vi "basic-reception.vi"(0 "Digital in":refnum<vi>, 1 "Cluster 5":T1, 2 "Lickometer":refnum<vi>, 3 "reference in":refnum<vi>, 5 "relative seconds":dbl, 7 "Cluster in":T2, 9 "Current Number Reception Licks":i32, 11 "Period":i64, 12 "Numeric 2":dbl, 13 "Numeric":dbl, 14 "Min Licks":i32) -> (4 "Cluster 4":T1, 6 "Cluster out":T2)   [LabVIEW 2015]
uses:
  <vilib>/Platform/TimedLoop/XDataNode/wakeup.ctl
  <vilib>/Platform/TimedLoop/XDataNode/XDNodeRunTimeDep.lvlib
  <vilib>/Platform/TimedLoop/XDataNode/nitl_modes.ctl
  <vilib>/Platform/TimedLoop/XDataNode/timing_clust.ctl
  <vilib>/platform/TimedLoop/XDataNode/XDataNode.xnode
  Device/Methods/Lickometer-Read.vi
  Rack/Methods/Rack-Refresh.vi
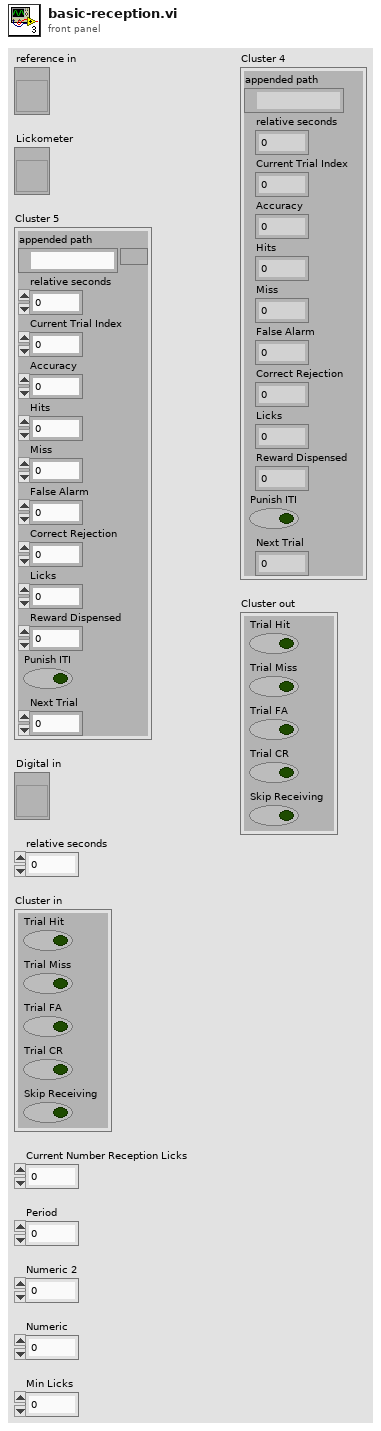
[diagram p1: front panel]
types:
  T1 = cluster{"appended path":path, "relative seconds":dbl, "Current Trial Index":i32, "Accuracy":dbl, "Hits":i32, "Miss":i32, "False Alarm":i32, "Correct Rejection":i32, "Licks":i32, "Reward Dispensed":dbl, "Punish ITI":bool, "Next Trial":i32}
  T2 = cluster{"Trial Hit":bool, "Trial Miss":bool, "Trial FA":bool, "Trial CR":bool, "Skip Receiving":bool}
  T3 = typedef "XDNodeRunTimeDep.lvlib/timing_clust.ctl" = cluster{"Expected End [f-1]":u64, "Actual End [f-1]":u64, "Finished Late? [f-1]":bool, "Expected End [i-1]":u64, "Actual End [i-1]":u64, "Finished Late? [i-1]":bool, "Expected Start [i]":u64, "Actual Start [i]":u64, "Expected Start [f]":u64, "Actual Start [f]":u64, "Source Name":string, "Structure Name":string, "Period":i64, "Deadline":i64, "Offset":i64, "Start":i64, "Priority":i32, "Timeout":i32, "Mode":T4, "Wakeup Reason":T5, "Error":errorcluster, "Source Type":string, "Secondary Source Type":string, "Global End Time":u64, "Global Start Time":u64, "Frame Duration":u64, "Iteration Duration":u64, "Assigned CPU":i32, "I/O Scan Engine Mode":u32}
  T4 = typedef "XDNodeRunTimeDep.lvlib/nitl_modes.ctl" = enum32{"No Change", "Process missed periods, maintain original phase", "Discard missed periods, maintain original phase", "Process missed periods, ignore original phase", "Discard missed periods, ignore original phase"}
  T5 = typedef "XDNodeRunTimeDep.lvlib/wakeup.ctl" = enum32{"Normal", "Aborted", "Asynchronous wakeup", "Timing source error", "Timed loop error", "Timeout"}
  T6 = typedef "InputData cluster.ctl" = cluster{"DigitalInput":T7}
  T7 = typedef "DigitalInput-DataCluster.ctl" = cluster{"Falling":bool[], "Rising":bool[], "State":bool[]}
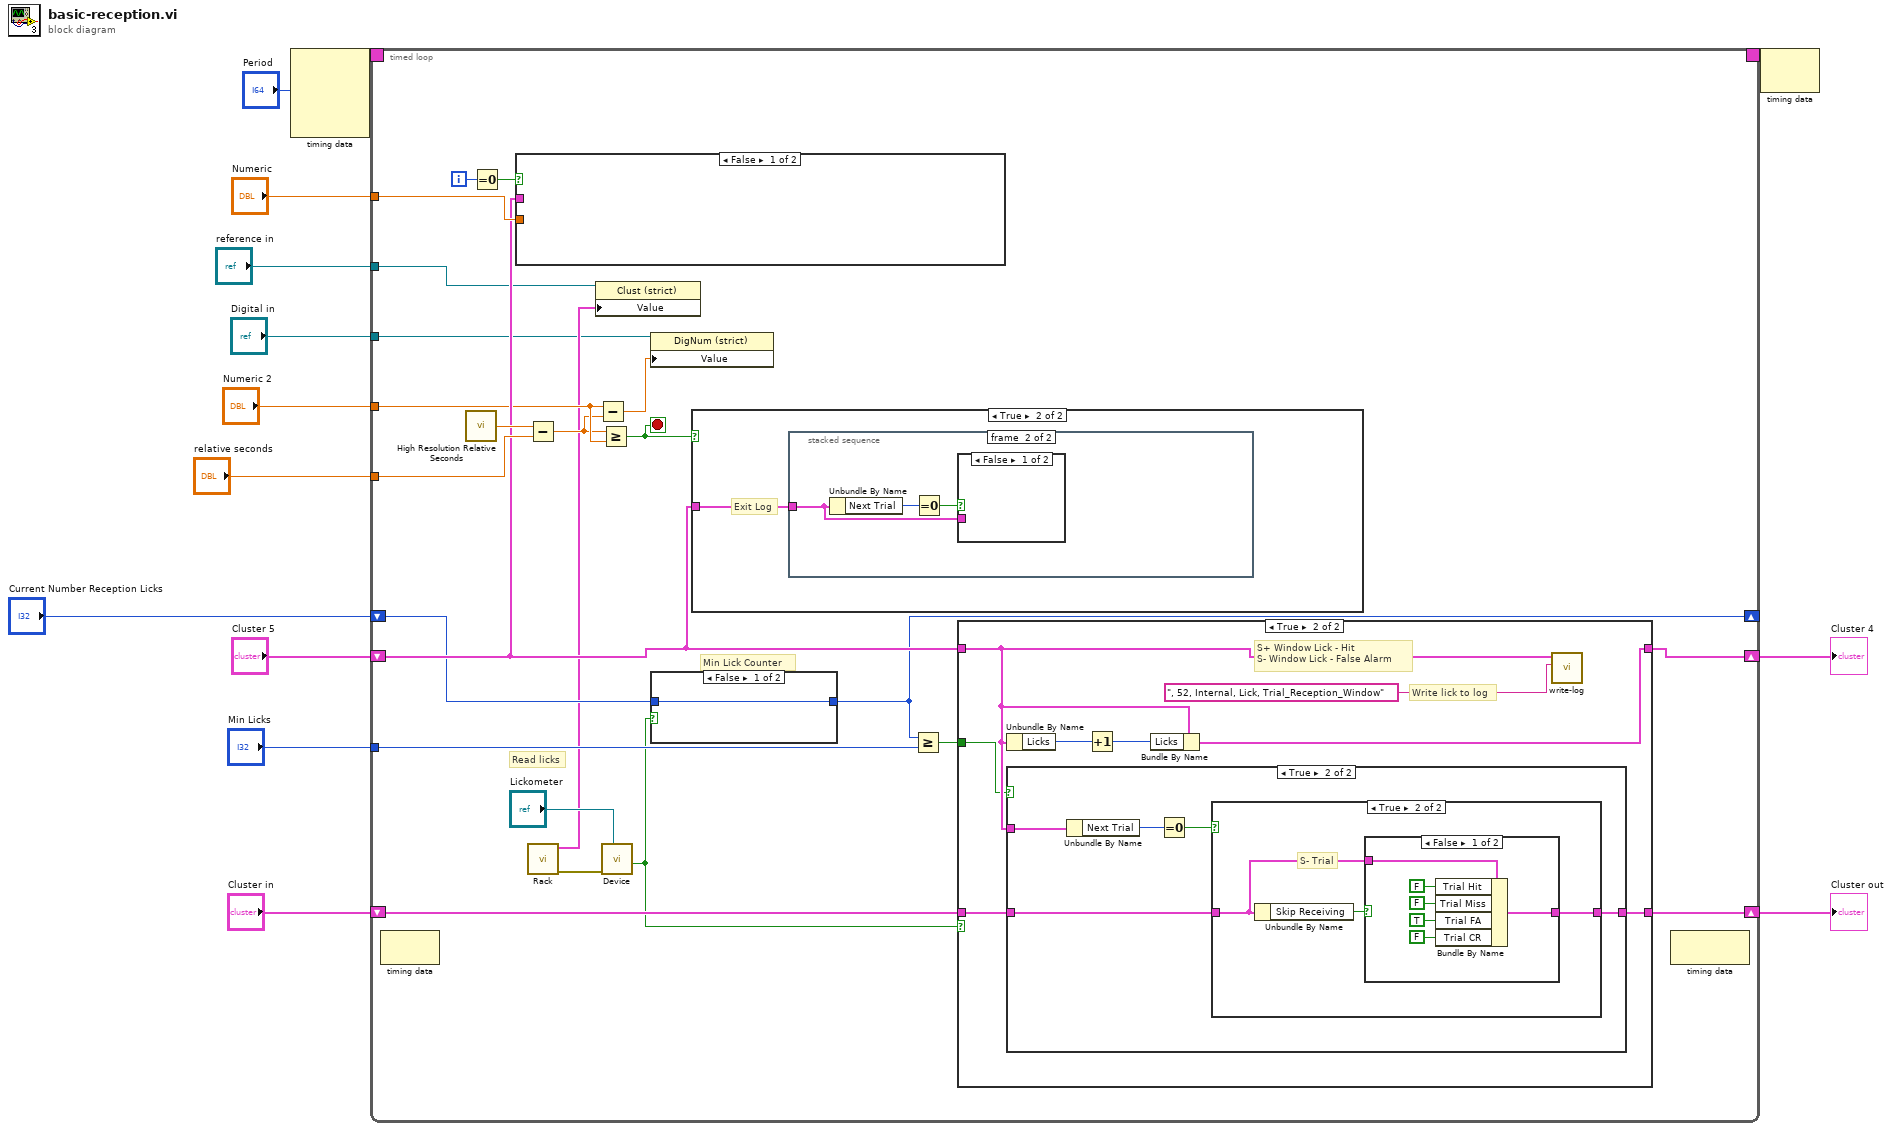
[diagram p0: block diagram]
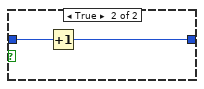
[diagram p2: hidden frame]
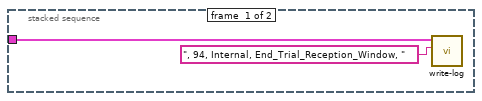
[diagram p4: hidden frame]
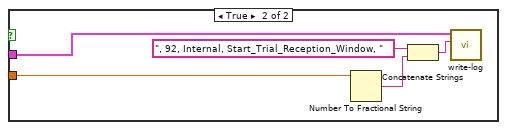
[diagram p6: hidden frame]
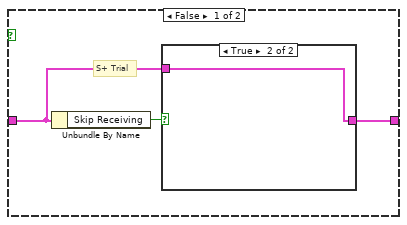
[diagram p9: hidden frame]
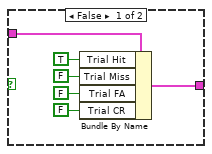
[diagram p10: hidden frame]
diagram:
  n1 = node-c288("Period") -> (w14:T3)  [unwired: 3 in]
  n2 = timed-loop {
    tunnel: "Numeric 2" -> [w20]
    tunnel: "relative seconds" -> [w35]
    shift-right: [w36] -> w9
    shift-left: "Cluster 5" -> [w28]
    tunnel: "Numeric" -> [w30]
    shift-right: [w33] -> w8
    shift-left: "Cluster in" -> [w34]
    shift-right: [w26] -> _
    shift-left: "Current Number Reception Licks" -> [w27]
    tunnel: "Min Licks" -> [w25]
    timing: w14 -> [_]
    timing-out: [_] -> w13
    tunnel: "Digital in" -> [w16]
    tunnel: "reference in" -> [w15]
    i -> [w32]
    stop <- w29 stop-if-true
    # "Min Lick Counter"
    # "Read licks"
    n3 = node-c288() -> ()  [unwired: 1 in, 1 out]
    n4 = call <vilib>:"High Resolution Relative Seconds.vi"() -> ("relative seconds"=w37:dbl)
    n5 = Equal To 0?(x=w32) -> (x = 0?=w31:bool)
    n6 = case shown="False" w31 {
      tunnel: w28 -> [_ w53]
      tunnel: w30 -> [_ w49]
      frame False {
      }
      frame True {
        n7 = Number To Fractional String(number=w49) -> (F-format string=w50:string)  [unwired: 3 in]
        n8 = Concatenate Strings(", 92, Internal, Start_Trial_Reception_Window, " ("text"), w50) -> (w52:string)
        n9 = call "write-log.vi"("Write Text"=w52, "Internal Cluster"=w53) -> ()  [unwired: 10 in]
      }
    }
    n10 = Subtract(x=w37, y=w35) -> (x-y=w19:dbl)
    n11 = call-poly "Rack.vi"() -> ("error out"=w23:errorcluster, "Data Cluster"=w17:T6)  [unwired: 10 in]
    n12 = property class="Clust (strict)"(reference=w15, "Value"=w17) -> ()  [unwired: 1 in, 2 out]
    n13 = Subtract(x=w20, y=w19) -> (x-y=w18:dbl)
    n14 = Greater Or Equal?(x=w19, y=w20) -> (x >= y?=w29:bool)
    n15 = call-poly "Device.vi"("Device reference"="Lickometer", "error in (no error)"=w23) -> ("Lick start?"=w22:bool)  [unwired: 7 in, 2 out]
    n16 = property class="DigNum (strict)"(reference=w16, "Value"=w18) -> ()  [unwired: 1 in, 2 out]
    n17 = case shown="False" w22 {
      tunnel: w27 -> [w40 w42]
      tunnel: [w40 w41] -> w26
      frame False {
      }
      frame True {
        n18 = Increment(x=w42) -> (x+1=w41:i32)
      }
    }
    n19 = case shown="True" w29 {
      tunnel: w28 -> [_ w43]
      frame False {
      }
      frame True {
        # "Exit Log"
        n20 = stacked-sequence {
          tunnel: w43 -> [w44 w48]
          frame #0 {
            n21 = call "write-log.vi"("Write Text"=", 94, Internal, End_Trial_Reception_Window, " ("text"), "Internal Cluster"=w44) -> ()  [unwired: 10 in]
          }
          frame #1 {
            n22 = Unbundle By Name(w48) -> ("Next Trial"=w47:i32)
            n23 = Equal To 0?(x=w47) -> (x = 0?=w46:bool)
            n24 = case shown="False" w46 {
              tunnel: w48 -> [_ _]
              frame False {
              }
              frame True {
              }
            }
          }
        }
      }
    }
    n25 = Greater Or Equal?(x=w26, y=w25) -> (x >= y?=w24:bool)
    n26 = case shown="True" w22 {
      tunnel: w28 -> [w55 w59]
      tunnel: [w55 w60] -> w36
      tunnel: w34 -> [w54 w58]
      tunnel: [w54 w57] -> w33
      tunnel: w24 -> [_ w56]
      frame False {
      }
      frame True {
        # "S+ Window Lick - Hit\nS- Window Lick - False Alarm"
        # "Write lick to log"
        n27 = Unbundle By Name(w59) -> ("Licks"=w62:i32)
        n28 = case shown="True" w56 {
          tunnel: w59 -> [_ w69]
          tunnel: w58 -> [w64 w66]
          tunnel: [w64 w65] -> w57
          frame False {
          }
          frame True {
            n29 = Unbundle By Name(w69) -> ("Next Trial"=w68:i32)
            n30 = Equal To 0?(x=w68) -> (x = 0?=w67:bool)
            n31 = case shown="True" w67 {
              tunnel: w66 -> [w71 w81]
              tunnel: [w70 w80] -> w65
              frame False {
                # "S+ Trial"
                n32 = Unbundle By Name(w71) -> ("Skip Receiving"=w72:bool)
                n33 = case shown="True" w72 {
                  tunnel: w71 -> [w74 w79]
                  tunnel: [w73 w79] -> w70
                  frame False {
                    n34 = Bundle By Name(cluster=w74, "Trial Hit"=TRUE, "Trial Miss"=FALSE, "Trial FA"=FALSE ("Trial CR"), "Trial CR"=FALSE ("Trial FA")) -> (w73:T2)
                  }
                  frame True {
                  }
                }
              }
              frame True {
                # "S- Trial"
                n35 = Unbundle By Name(w81) -> ("Skip Receiving"=w82:bool)
                n36 = case shown="False" w82 {
                  tunnel: w81 -> [w84 w89]
                  tunnel: [w83 w89] -> w80
                  frame False {
                    n37 = Bundle By Name(cluster=w84, "Trial Hit"=FALSE, "Trial Miss"=FALSE, "Trial FA"=TRUE ("Trial CR"), "Trial CR"=FALSE ("Trial FA")) -> (w83:T2)
                  }
                  frame True {
                  }
                }
              }
            }
          }
        }
        n38 = Increment(x=w62) -> (x+1=w61:i32)
        n39 = Bundle By Name(cluster=w59, "Licks"=w61) -> (w60:T1)
        n40 = call "write-log.vi"("Write Text"=", 52, Internal, Lick, Trial_Reception_Window" ("text"), "Internal Cluster"=w59) -> ()  [unwired: 10 in]
      }
    }
    n41 = node-c288() -> ()  [unwired: 1 in, 1 out]
  }
  "Cluster 4" <- w9
  "Cluster out" <- w8
  n42 = node-c288(w13) -> ()  [unwired: 1 out]
